vi "Configure Ref Clock Source.vi"(8 "error in (no error)":errorcluster, 9 "reference clock source (Internal)":i32(ring) items=["Internal"=0, "External"=1, "RTSI Clock"=101], 11 "CS++Fgen in":refnum<class "CS++Fgen.lvclass">) -> (0 "error out":errorcluster, 3 "CS++Fgen out":refnum<class "CS++Fgen.lvclass">)   [LabVIEW 2013, in "CS++Fgen.lvlib" / "CS++Fgen.lvclass"]
doc: "This VI configures the function generator's reference clock source. The function generator uses the reference clock to derive frequencies and sample rates when generating output."
uses:
  CS++Fgen.lvclass
  Core/Classes/CS++ProcessVariables/ProcessVariable/PV.lvclass
  Core/Classes/CS++ProcessVariables/ProcessVariable/PV.lvclass/PV.ctl
  CS++Fgen.lvclass/CS++Fgen.ctl
  Core/Classes/CS++ProcessVariables/PVConnection/PVConnection.lvclass
  Core/Classes/CS++ProcessVariables/ProcessVariable/Write Data.vi
  Core/Classes/CS++ProcessVariables/ProcessVariable/Write Timestamp.vi
  Core/Classes/CS++ProcessVariables/ProcessVariable/Write Quality.vi
  Core/Classes/CS++ProcessVariables/ProcessVariable/Write status.vi
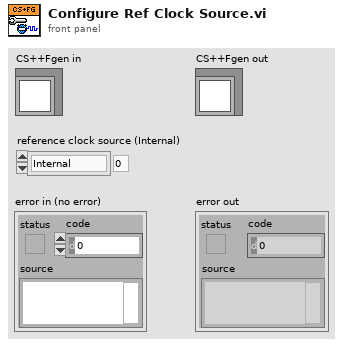
[diagram p1: front panel]
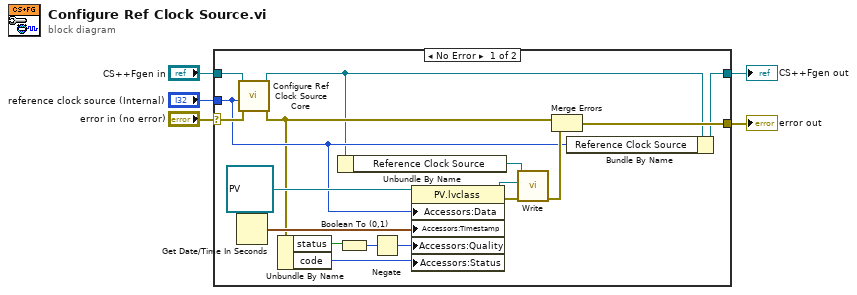
[diagram p0: block diagram]
diagram:
  n1 = case shown="No Error" "error in (no error)" {
    selector: "error in (no error)" -> [w21 w24]
    tunnel: [w8 w24] -> w4
    tunnel: [w6 w23] -> w2
    tunnel: "CS++Fgen in" -> [w22 w23]
    tunnel: "reference clock source (Internal)" -> [w10 _]
    frame No Error {
      n2 = Get Date/Time In Seconds() -> (seconds since 1Jan1904=w20:timestamp)
      n3 = call-dynamic "Configure Ref Clock Source Core.vi"("error in (no error)"=w21, "reference clock source (Internal)"=w10, "CS++Fgen in"=w22) -> ("error out"=w9:errorcluster, "CS++Fgen out"=w7:refnum<class "CS++Fgen.lvclass">)  [unwired: 7 in]
      n4 = Unbundle By Name(w9) -> ("status"=w15:bool, "code"=w13:i32)
      n5 = Unbundle By Name(w7) -> ("Reference Clock Source"=w11:refnum<class "PVConnection.lvclass">)
      n6 = Boolean To (0,1)(Boolean=w15) -> (0, 1=w14:i16)
      n7 = Negate(x=w14) -> (-x=w12:i16)
      n8 = property class="PV.lvclass"(reference=refnum<class "PV.lvclass"> refnum ("PV"), "Accessors:Data"=w10, "Accessors:Timestamp"=w20, "Accessors:Quality"=w12, "Accessors:Status"=w13) -> (reference out=w17:refnum<class "PV.lvclass">, error out=w18:errorcluster)  [unwired: 1 in]
      n9 = call-dynamic "Write.vi"("error in (no error)"=w18, "PV"=w17, "PVConnection in"=w11) -> ("error out"=w16:errorcluster)  [unwired: 7 in, 1 out]
      n10 = Merge Errors(w9, w16) -> (w8:errorcluster)
      n11 = Bundle By Name(cluster=w7, "Reference Clock Source"=w10) -> (w6:refnum<class "CS++Fgen.lvclass">)
    }
    frame Error {
    }
  }
  "error out" <- w4
  "CS++Fgen out" <- w2
